vi "registers to data.vi"(9 "specifications":T1[](array[typedef]), 10 "registers":u16[](array[numeric]), 11 "allocation":T3) -> (3 "data table":T3)   [LabVIEW 2013, in "Modbus Slave runtime.lvclass"]
uses:
  Modbus Slave runtime.lvclass
  <vilib>/NI/Tag Bus/table/data table.ctl
  data mapping elements.ctl
  <vilib>/NI/Tag Bus/tag/Data Type.ctl
  <vilib>/NI/Tag Bus/table/data polymorphs/write one/write Double.vi
  <vilib>/NI/Tag Bus/table/data polymorphs/write one/write Single.vi
  <vilib>/NI/Tag Bus/table/data polymorphs/write one/write I64.vi
  <vilib>/NI/Tag Bus/table/data polymorphs/write one/write U64.vi
  <vilib>/NI/Tag Bus/table/data polymorphs/write one/write I32.vi
  <vilib>/NI/Tag Bus/table/data polymorphs/write one/write U32.vi
  <vilib>/NI/Tag Bus/table/data polymorphs/write one/write I16.vi
  <vilib>/NI/Tag Bus/table/data polymorphs/write one/write U16.vi
  <vilib>/NI/Tag Bus/table/data polymorphs/write one/write I8.vi
  <vilib>/NI/Tag Bus/table/data polymorphs/write one/write Boolean.vi
  <vilib>/NI/Tag Bus/table/data table.lvlib
  <vilib>/NI/Tag Bus/tag/tag descriptor.lvclass
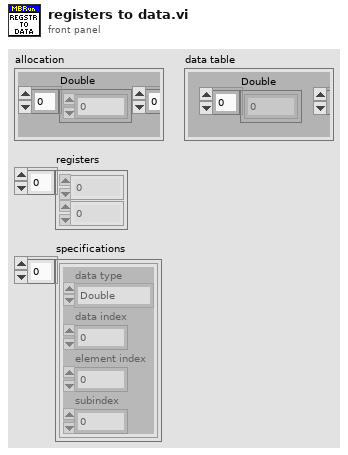
[diagram p1: front panel]
types:
  T1 = typedef "Modbus Slave runtime.lvclass/data mapping elements.ctl" = cluster{"data type":T2, "data index":i32, "element index":i32, "subindex":i32}
  T2 = typedef "tag bus.lvlib/tag descriptor.lvclass/Data Type.ctl" = enum16{"Double", "Single", "I64", "I32", "I16", "I8", "U64", "U32", "U16", "U8", "Boolean", "String", "Array of Double", "Array of Single", "Array of I64", "Array of I32", "Array of I16", "Array of I8", "Array of U64", "Array of U32", "Array of U16", "Array of U8", "Array of Boolean", "Array of String"}
  T3 = typedef "tag bus.lvlib/data table.lvlib/data table.ctl" = cluster{"Double":dbl[], "Single":sgl[], "I64":i64[], "I32":i32[], "I16":i16[], "I8":i8[], "U64":u64[], "U32":u32[], "U16":u16[], "U8":u8[], "Boolean":bool[], "String":string[], "Array of Double":cluster{"DBL Array":dbl[]}[], "Array of Single":cluster{"SGL Array":sgl[]}[], "Array of I64":cluster{"I64 Array":i64[]}[], "Array of I32":cluster{"I32 Array":i32[]}[], "Array of I16":cluster{"I16 Array":i16[]}[], "Array of I8":cluster{"I8 Array":i8[]}[], "Array of U64":cluster{"U64 Array":u64[]}[], "Array of U32":cluster{"U32 Array":u32[]}[], "Array of U16":cluster{"U16 Array":u16[]}[], "Array of U8":cluster{"U8 Array":u8[]}[], "Array of Boolean":cluster{"Boolean Array":bool[]}[], "Array of String":cluster{"String Array":string[]}[]}
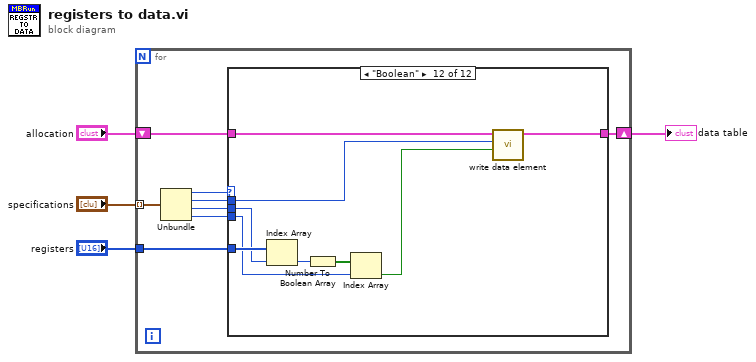
[diagram p0: block diagram]
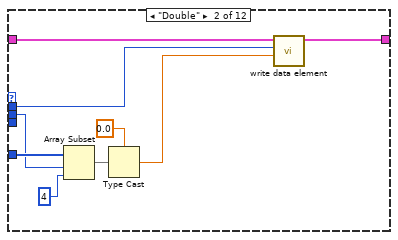
[diagram p3: hidden frame]
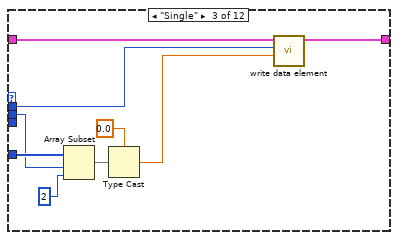
[diagram p4: hidden frame]
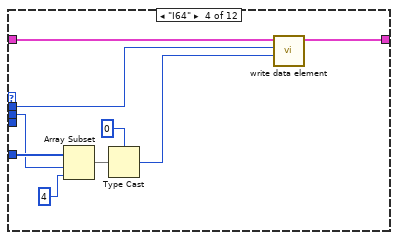
[diagram p5: hidden frame]
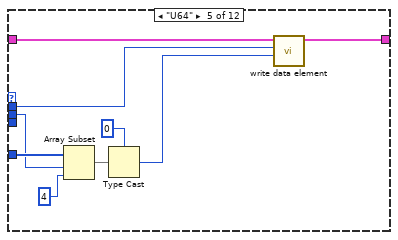
[diagram p6: hidden frame]
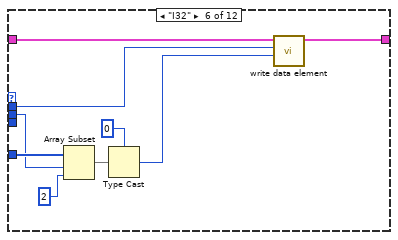
[diagram p7: hidden frame]
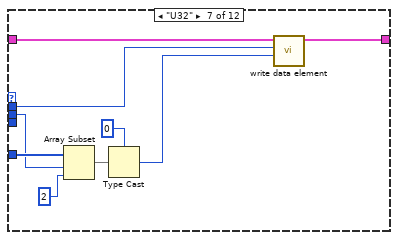
[diagram p8: hidden frame]
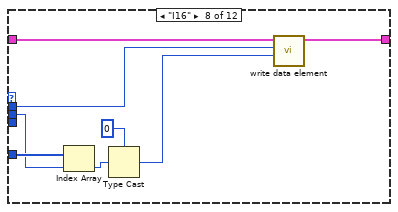
[diagram p9: hidden frame]
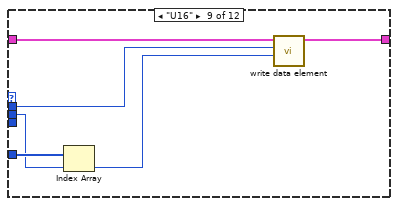
[diagram p10: hidden frame]
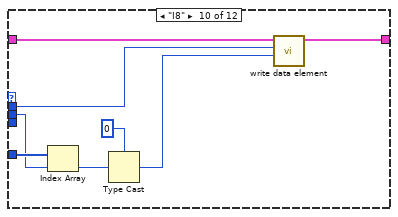
[diagram p11: hidden frame]
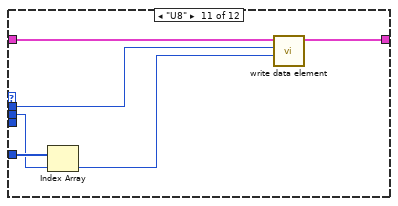
[diagram p12: hidden frame]
diagram:
  n1 = for {
    shift-right: [w9] -> w3
    shift-left: "allocation" -> [w10]
    tunnel: "registers" -> [w8]
    tunnel: "specifications" -> [w12] mode=indexing
    n2 = Unbundle(w12) -> ("data type"=w11:T2, "data index"=w7:i32, "element index"=w5:i32, "subindex"=w6:i32)
    n3 = case shown="\"Boolean\"" w11 {
      tunnel: w10 -> [w13 w22 w31 w40 w49 w58 w67 w75 w81 w89 w95 w104]
      tunnel: [w13 w21 w30 w39 w48 w57 w66 w74 w80 w88 w94 w103] -> w9
      tunnel: w5 -> [_ w18 w27 w36 w45 w54 w63 w72 w78 w86 w92 w101]
      tunnel: w8 -> [_ w20 w29 w38 w47 w56 w65 w73 w79 w87 w93 w102]
      tunnel: w7 -> [_ w17 w26 w35 w44 w53 w62 w71 w77 w85 w91 w100]
      tunnel: w6 -> [_ _ _ _ _ _ _ _ _ _ _ w96]
      frame Default {
      }
      frame "Double" {
        n4 = Array Subset(array=w20, index=w18, length=4 ("x")) -> (w16:u16[])
        n5 = Type Cast(type=0.0, x=w16) -> (*(type *) &x=w14:dbl)
        n6 = call-poly <vilib>:"write data element.vi"("value"=w14, "index"=w17, "data table in"=w22) -> ("data table out"=w21:T3)  [unwired: 8 in]
      }
      frame "Single" {
        n7 = Array Subset(array=w29, index=w27, length=2 ("x")) -> (w25:u16[])
        n8 = Type Cast(type=sgl 0.0, x=w25) -> (*(type *) &x=w23:sgl)
        n9 = call-poly <vilib>:"write data element.vi"("value"=w23, "index"=w26, "data table in"=w31) -> ("data table out"=w30:T3)  [unwired: 8 in]
      }
      frame "I64" {
        n10 = Array Subset(array=w38, index=w36, length=4 ("x")) -> (w34:u16[])
        n11 = Type Cast(type=i64 0, x=w34) -> (*(type *) &x=w32:i64)
        n12 = call-poly <vilib>:"write data element.vi"("value"=w32, "index"=w35, "data table in"=w40) -> ("data table out"=w39:T3)  [unwired: 8 in]
      }
      frame "U64" {
        n13 = Array Subset(array=w47, index=w45, length=4 ("x")) -> (w43:u16[])
        n14 = Type Cast(type=u64 0, x=w43) -> (*(type *) &x=w41:u64)
        n15 = call-poly <vilib>:"write data element.vi"("value"=w41, "index"=w44, "data table in"=w49) -> ("data table out"=w48:T3)  [unwired: 8 in]
      }
      frame "I32" {
        n16 = Array Subset(array=w56, index=w54, length=2 ("x")) -> (w52:u16[])
        n17 = Type Cast(type=0, x=w52) -> (*(type *) &x=w50:i32)
        n18 = call-poly <vilib>:"write data element.vi"("value"=w50, "index"=w53, "data table in"=w58) -> ("data table out"=w57:T3)  [unwired: 8 in]
      }
      frame "U32" {
        n19 = Array Subset(array=w65, index=w63, length=2 ("x")) -> (w61:u16[])
        n20 = Type Cast(type=u32 0, x=w61) -> (*(type *) &x=w59:u32)
        n21 = call-poly <vilib>:"write data element.vi"("value"=w59, "index"=w62, "data table in"=w67) -> ("data table out"=w66:T3)  [unwired: 8 in]
      }
      frame "I16" {
        n22 = Index Array(array=w73, index=w72) -> (element=w70:u16)
        n23 = Type Cast(type=i16 0, x=w70) -> (*(type *) &x=w68:i16)
        n24 = call-poly <vilib>:"write data element.vi"("value"=w68, "index"=w71, "data table in"=w75) -> ("data table out"=w74:T3)  [unwired: 8 in]
      }
      frame "U16" {
        n25 = Index Array(array=w79, index=w78) -> (element=w76:u16)
        n26 = call-poly <vilib>:"write data element.vi"("value"=w76, "index"=w77, "data table in"=w81) -> ("data table out"=w80:T3)  [unwired: 8 in]
      }
      frame "I8" {
        n27 = Index Array(array=w87, index=w86) -> (element=w84:u16)
        n28 = Type Cast(type=i8 0, x=w84) -> (*(type *) &x=w82:i8)
        n29 = call-poly <vilib>:"write data element.vi"("value"=w82, "index"=w85, "data table in"=w89) -> ("data table out"=w88:T3)  [unwired: 8 in]
      }
      frame "U8" {
        n30 = Index Array(array=w93, index=w92) -> (element=w90:u16)
        n31 = call-poly <vilib>:"write data element.vi"("value"=w90, "index"=w91, "data table in"=w95) -> ("data table out"=w94:T3)  [unwired: 8 in]
      }
      frame "Boolean" {
        n32 = Index Array(array=w102, index=w101) -> (element=w99:u16)
        n33 = Number To Boolean Array(number=w99) -> (Boolean array=w98:bool[])
        n34 = Index Array(array=w98, index=w96) -> (element=w97:bool)
        n35 = call-poly <vilib>:"write data element.vi"("value"=w97, "index"=w100, "data table in"=w104) -> ("data table out"=w103:T3)  [unwired: 8 in]
      }
    }
  }
  "data table" <- w3
